vi "GetElement(Single).vi"(7 "Qualified Name":string, 8 "error in (no error)":errorcluster, 10 "Key":string, 11 "SMOConfigManagerCollection in":refnum<class "ConfigManagerCollection.lvclass">) -> (0 "error out":errorcluster, 1 "found":bool, 2 "Value":string, 3 "SMOConfigManagerCollection out":refnum<class "ConfigManagerCollection.lvclass">)   [LabVIEW 2013, in "SMOConfig.lvlib" / "ConfigManagerCollection.lvclass"]
uses:
  ConfigManagerCollection.lvclass
  Manager/ConfigManager.lvclass
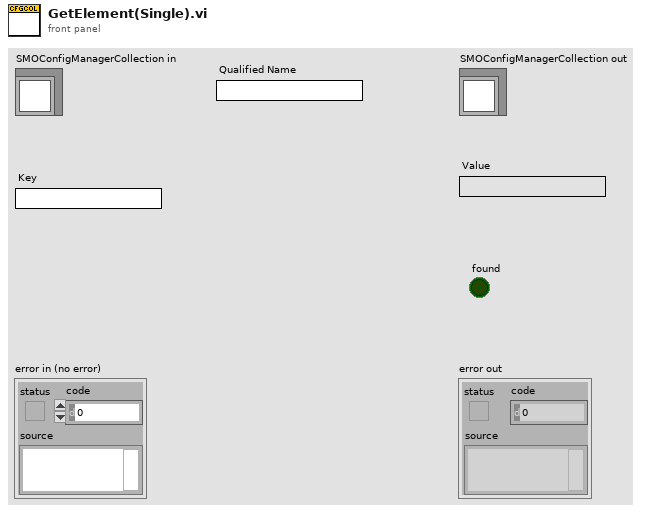
[diagram p1: front panel]
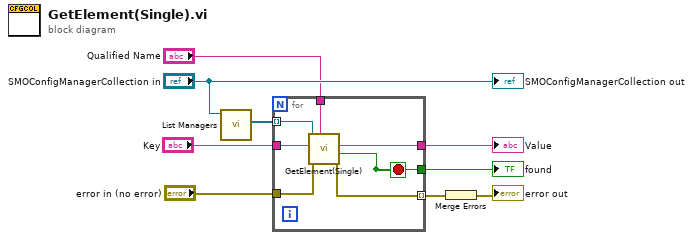
[diagram p0: block diagram]
diagram:
  n1 = call-dynamic "List Managers.vi"("SMOConfigManagerCollection in"="SMOConfigManagerCollection in") -> ("List"=w8:refnum<class "ConfigManager.lvclass">[])  [unwired: 9 in, 1 out]
  n2 = for {
    tunnel: w8 -> [w11] mode=indexing
    tunnel: "Key" -> [w16]
    tunnel: "error in (no error)" -> [w15]
    tunnel: [w14] -> w5 mode=indexing
    tunnel: [w13] -> w3
    tunnel: [w12] -> w2
    tunnel: "Qualified Name" -> [w10]
    stop <- w13 stop-if-true
    n3 = call-dynamic "GetElement(Single).vi"("Qualified Name"=w10, "error in (no error)"=w15, "Key"=w16, "SMOConfigManager in"=w11) -> ("error out"=w14:errorcluster, "found"=w13:bool, "Value"=w12:string)  [unwired: 4 in, 1 out]
  }
  "Value" <- w2
  "found" <- w3
  n4 = Merge Errors(w5) -> (→"error out":errorcluster)
  "SMOConfigManagerCollection out" <- "SMOConfigManagerCollection in"
